vi "get rate.vi"(8 "error in":errorcluster, 11 "timing source in":refnum<class "scan engine timing source.lvclass">) -> (0 "error out":errorcluster, 2 "period (ns)":i64, 3 "timing source out":refnum<class "scan engine timing source.lvclass">)   [LabVIEW 2013, in "scan engine timing source.lvclass"]
doc: "Returns the rate of the clock used by the selected timing source. This rate is the period measured in nanoseconds."
uses:
  scan engine timing source.lvclass
  scan engine timing source.lvclass/scan engine timing source.ctl
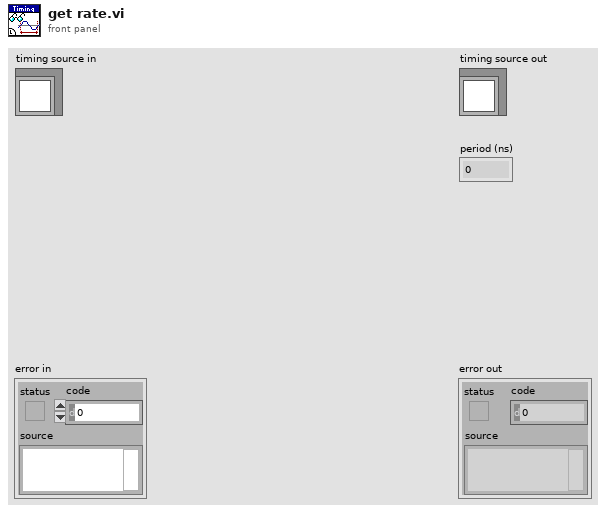
[diagram p1: front panel]
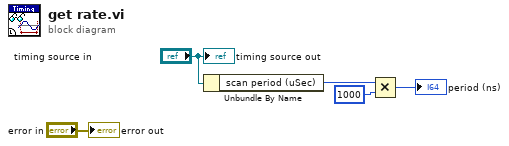
[diagram p0: block diagram]
diagram:
  n1 = Unbundle By Name("timing source in") -> ("scan period (uSec)"=w3:u32)
  n2 = Multiply(x=w3, y=i64 1000) -> (x*y=→"period (ns)":i64)
  "error out" <- "error in"
  "timing source out" <- "timing source in"
